vi "sqlbackup.vi"(8 "error in (no error)":errorcluster caption="错误输入（无错误）") -> (0 "error out":errorcluster caption="错误输出")   [LabVIEW 2016, in "数据查询.lvlib"]
uses:
  var/holding var.vi
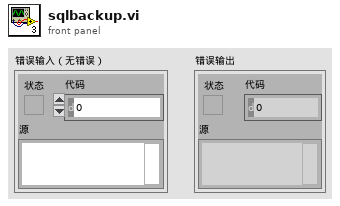
[diagram p1: front panel]
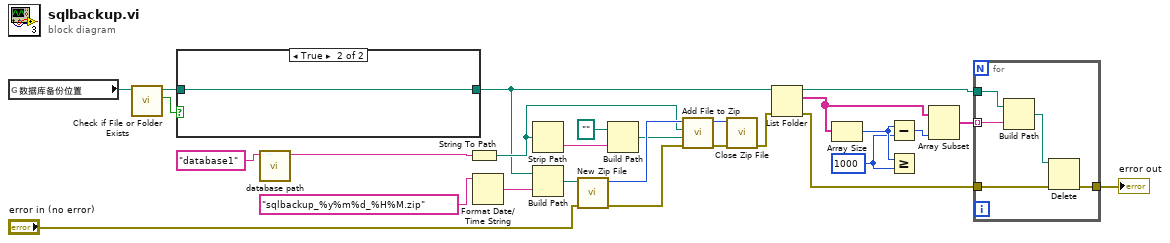
[diagram p0: block diagram]
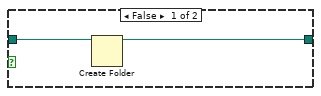
[diagram p2: hidden frame]
diagram:
  w7 = 1000 ("y")
  n1 = global read "holding var.vi" "数据库备份位置"() -> (w14:path)
  n2 = call <vilib>:"Check if File or Folder Exists.vi"("path"=w14) -> ("file or folder exists?"=w13:bool, "dup path"=w12:path)  [unwired: 8 in, 1 out]
  n3 = case shown="True" w13 {
    tunnel: w12 -> [w29 w30]
    tunnel: [w28 w30] -> w10
    frame False {
      n4 = Create Folder(path (use dialog)=w29) -> (created path=w28:path)  [unwired: 2 in, 2 out]
    }
    frame True {
    }
  }
  n5 = call "database path.vi"("database"="database1") -> ("Path out"=w26:string)  [unwired: 9 in, 1 out]
  n6 = String To Path(string=w26) -> (path=w18:path)
  n7 = Format Date/Time String(time format string (%c)="sqlbackup_%y%m%d_%H%M.zip" ("时间格式字符串(%c)")) -> (date/time string=w20:string)  [unwired: 2 in]
  n8 = Strip Path(path=w18) -> (name=w17:string)  [unwired: 1 out]
  n9 = Build Path(base path=w10, name or relative path=w20) -> (appended path=w19:path)
  n10 = call <vilib>:"New Zip File.vi"("error in (no error)"="error in (no error)", "target"=w19) -> ("error out"=w23:errorcluster, "zip file out"=w25:i64)  [unwired: 3 in, 1 out]
  n11 = Build Path(base path=path "" ("基路径"), name or relative path=w17) -> (appended path=w15:path)
  n12 = call <vilib>:"Add File to Zip.vi"("error in (no error)"=w23, "destination path in zip"=w15, "source file path"=w18, "zip file in"=w25) -> ("error out"=w22:errorcluster, "zip file out"=w24:i64)  [unwired: 6 in]
  n13 = call <vilib>:"Close Zip File.vi"("error in (no error)"=w22, "zip file in"=w24) -> ("error out"=w3:errorcluster)  [unwired: 5 in]
  n14 = List Folder(path=w10, error in=w3) -> (path out=w4:path, filenames=w9:string[], error out=w2:errorcluster)  [unwired: 2 in, 1 out]
  n15 = Array Size(array=w9) -> (size(s)=w8:i32)
  n16 = Subtract(x=w8, y=w7) -> (x-y=w6:i32)
  n17 = Greater Or Equal?(x=w8, y=w7) -> ()  [unwired: 1 out]
  n18 = Array Subset(array=w9, length=w6) -> (w5:string[])  [unwired: 1 in]
  n19 = for {
    tunnel: w5 -> [w34] mode=indexing
    tunnel: w4 -> [w35]
    tunnel: w2 -> [w32]
    tunnel: [w31] -> w1
    n20 = Build Path(base path=w35, name or relative path=w34) -> (appended path=w33:path)
    n21 = Delete(path (use dialog)=w33, error in=w32) -> (error out=w31:errorcluster)  [unwired: 3 in, 2 out]
  }
  "error out" <- w1
